vi "Read Operator Joystick.vi"   [LabVIEW 2020]
uses:
  <vilib>/Rock Robotics/WPI/Utilities/WPI_GetSetVariantRefNum.vi
  Framework/Robot Global Data.vi
  <vilib>/Rock Robotics/Network Tables/NT Write Numeric Array.vi
  <vilib>/Rock Robotics/Network Tables/NT Write Boolean Array.vi
types:
  T1 = enum16{"0", "1", "2", "3", "4", "5", "6", "7", "8", "9", "10", "11"}
  T2 = typedef "WPI_JoystickDevRef.ctl" = cluster{"Device":T3}
  T3 = typedef "WPI_JoystickDeviceEnum.ctl" = enum16{"USB 0", "USB 1", "USB 2", "USB 3", "USB 4", "USB 5"}
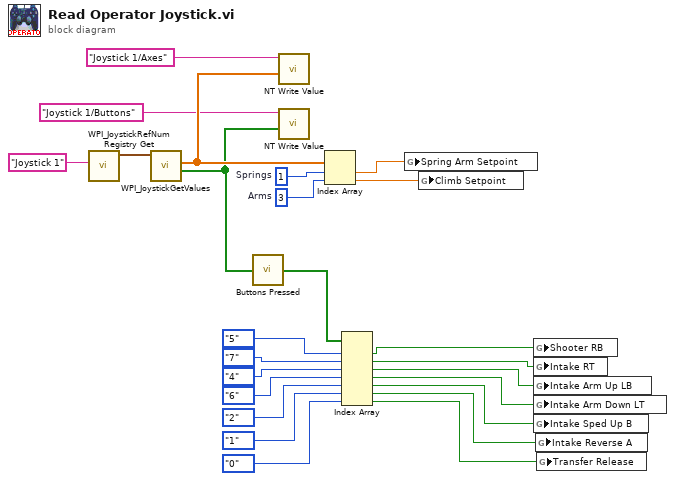
[diagram p0: block diagram]
diagram:
  w22 = 3  # Arms
  w23 = 1  # Springs
  n1 = call <vilib>:"WPI_JoystickRefNum Registry Get.vi"("refnum name"="Joystick 1") -> ("JoystickDevRef"=w25:T2)  [unwired: 9 in, 1 out]
  n2 = call <vilib>:"WPI_JoystickGetValues.vi"("JoystickDevRef"=w25) -> ("Buttons"=w20:bool[], "Axes"=w21:dbl[])  [unwired: 6 in, 3 out]
  n3 = call "Buttons Pressed.vi"("Button Values"=w20) -> ("Button Presses"=w19:bool[])
  n4 = call-poly <vilib>:"NT Write Value.vi"("Numeric Array"=w21, "Name"="Joystick 1/Axes") -> ()  [unwired: 9 in, 1 out]
  n5 = call-poly <vilib>:"NT Write Value.vi"("Boolean Array"=w20, "Name"="Joystick 1/Buttons") -> ()  [unwired: 9 in, 1 out]
  n6 = Index Array(array=w21, index #1=w23, index #2=w22) -> (element #1=w18:dbl, element #2=w17:dbl)
  n7 = Index Array(array=w19, index #1=T1."5", index #2=T1."7", index #3=T1."4", index #4=T1."6", index #5=T1."2", index #6=T1."1", index #7=T1."0") -> (element #1=w12:bool, element #2=w11:bool, element #3=w10:bool, element #4=w9:bool, element #5=w7:bool, element #6=w4:bool, element #7=w2:bool)
  n8 = global write "Robot Global Data.vi" "Spring Arm Setpoint"(w18) -> ()
  n9 = global write "Robot Global Data.vi" "Climb Setpoint"(w17) -> ()
  n10 = global write "Robot Global Data.vi" "Shooter RB"(w12) -> ()
  n11 = global write "Robot Global Data.vi" "Intake RT"(w11) -> ()
  n12 = global write "Robot Global Data.vi" "Intake Arm Up LB"(w10) -> ()
  n13 = global write "Robot Global Data.vi" "Intake Arm Down LT"(w9) -> ()
  n14 = global write "Robot Global Data.vi" "Intake Sped Up B"(w7) -> ()
  n15 = global write "Robot Global Data.vi" "Intake Reverse A"(w4) -> ()
  n16 = global write "Robot Global Data.vi" "Transfer Release"(w2) -> ()
